vi "Od_Lokal_PH.vi"() -> ()   [LabVIEW 2021]
panel:
  out "Proces 2:nr pêtli":i32
  in  "stop":bool
  out "Proces 1:nr pêtli":i32
  in  "CzyStop?":bool
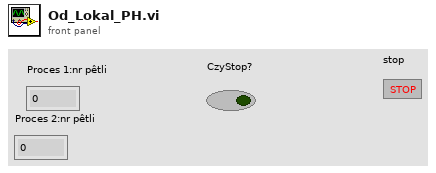
[diagram p1: front panel]
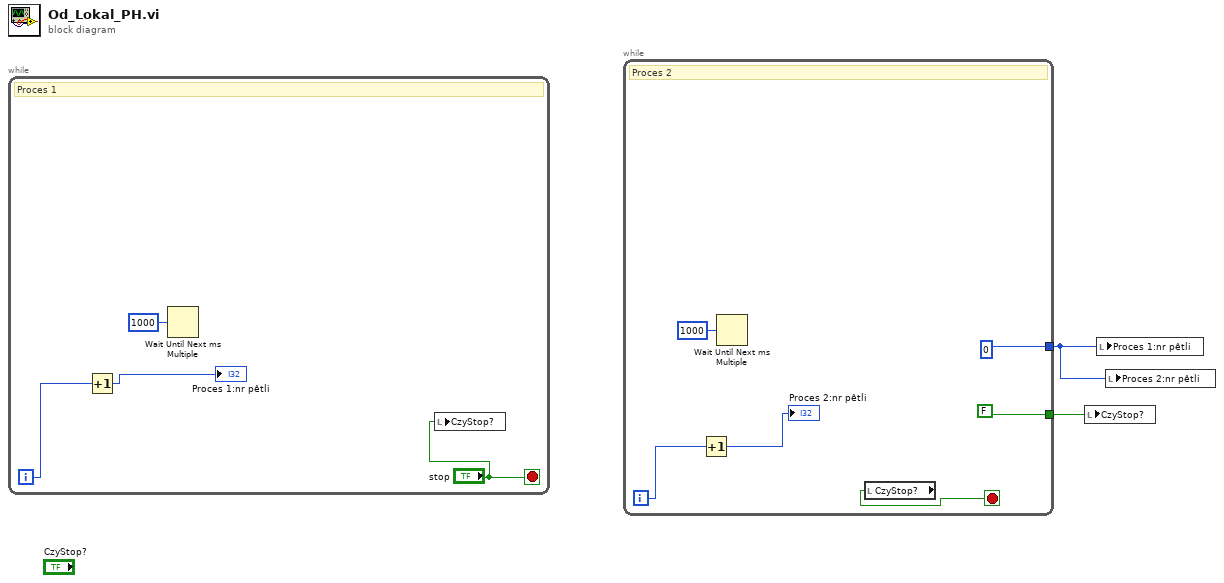
[diagram p0: block diagram]
diagram:
  n1 = while {
    i -> [w5]
    stop <- "stop" stop-if-true
    # "Proces 1"
    n2 = Increment(x=w5) -> (x+1=→"Proces 1:nr pêtli":i32)
    n3 = Wait Until Next ms Multiple(millisecond multiple=u32 1000) -> ()  [unwired: 1 out]
    n4 = local write "CzyStop?"("stop") -> ()
  }
  n5 = while {
    tunnel: [0] -> w2
    tunnel: [FALSE] -> w1
    i -> [w10]
    stop <- w9 stop-if-true
    # "Proces 2"
    n6 = Increment(x=w10) -> (x+1=→"Proces 2:nr pêtli":i32)
    n7 = Wait Until Next ms Multiple(millisecond multiple=u32 1000) -> ()  [unwired: 1 out]
    n8 = local read "CzyStop?"() -> (w9:bool)
  }
  n9 = local write "CzyStop?"(w1) -> ()
  n10 = local write "Proces 1:nr pêtli"(w2) -> ()
  n11 = local write "Proces 2:nr pêtli"(w2) -> ()
